vi "USBInterfaceFetch.vi"() -> ()   [LabVIEW 2022 SP3]
uses:
  be0127c4-6358-4ac6-84a7-134a79eb8395.vi
panel:
  in  "Ring":u16(ring) items=["Initialize Pump"=2, "Pump Status"=1, "Interface Only"=0]
  out "read buffer":string
  out "error out":errorcluster
  out "Interface Description":string
  in  "VISA resource name":refnum<visa-resource-name>
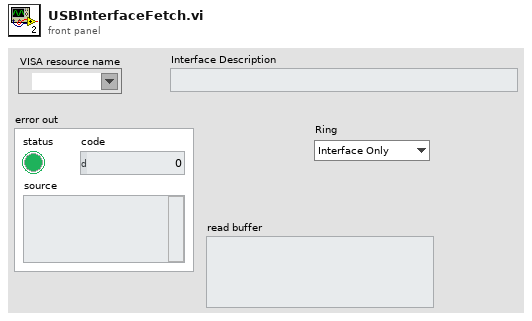
[diagram p1: front panel]
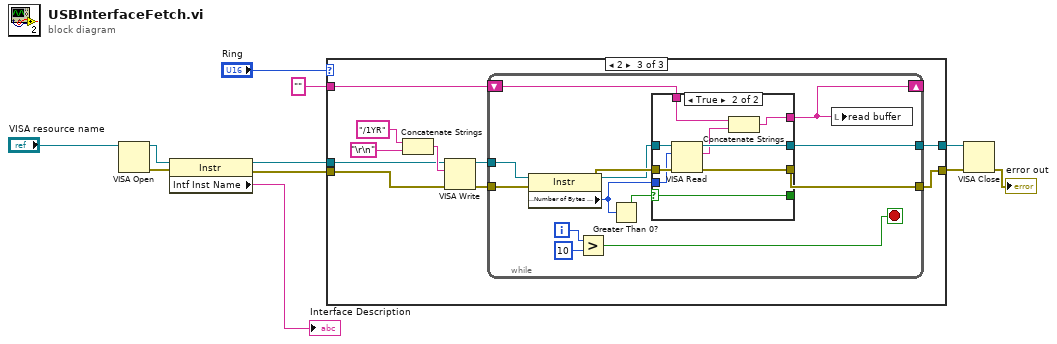
[diagram p0: block diagram]
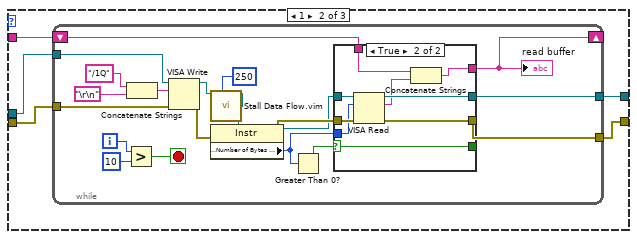
[diagram p3: hidden frame]
diagram:
  n1 = VISA Open(VISA resource name="VISA resource name") -> (VISA resource name=w11:refnum<visa-resource-name>, error out=w9:errorcluster)  [unwired: 4 in]
  n2 = property class="Instr"(reference=w11, error in=w9) -> (reference out=w6:refnum<visa-resource-name>, error out=w8:errorcluster, "Intf Inst Name"=→"Interface Description":string)
  n3 = case shown="2" "Ring" {
    tunnel: w8 -> [w12 w16 w55]
    tunnel: w6 -> [w13 w15 w54]
    tunnel: [w13 w18 w61] -> w4
    tunnel: [w12 w17 w60] -> w3
    tunnel: "" -> [_ w14 w59]
    frame 0, Default {
    }
    frame 1 {
      n4 = while {
        tunnel: [w34] -> w18
        tunnel: [w33] -> w17
        tunnel: w16 -> [w27]
        tunnel: w15 -> [w26]
        shift-right: [w20] -> _
        shift-left: w14 -> [w21]
        i -> [w32]
        stop <- w19 stop-if-true
        n5 = Greater?(x=w32, y=10) -> (0:w19:bool)
        n6 = Concatenate Strings("/1Q" ("write buffer"), "\r\n") -> (w30:string)
        n7 = VISA Write(VISA resource name=w26, write buffer=w30, error in (no error)=w27) -> (VISA resource name out=w23:refnum<visa-resource-name>, error out=w25:errorcluster)  [unwired: 1 out]
        n8 = call "Stall Data Flow.vim"("value in"=w23, "milliseconds to wait"=u32 250) -> ("value out"=w22:refnum<visa-resource-name>)  [unwired: 1 out]
        n9 = property class="Instr"(reference=w22, error in=w25) -> (reference out=w35:refnum<visa-resource-name>, error out=w36:errorcluster, "Serial Settings:Number of Bytes at Serial Port"=w38:u32)
        n10 = Greater Than 0?(x=w38) -> (x > 0?=w37:bool)
        n11 = case shown="True" w37 {
          selector: w37 -> [w40 w46]
          tunnel: w35 -> [w42 w51]
          tunnel: [w42 w50] -> w34
          tunnel: w36 -> [w41 w49]
          tunnel: [w41 w48] -> w33
          tunnel: w38 -> [_ w47]
          tunnel: [w40 w46] -> _
          tunnel: w21 -> [w39 w44]
          tunnel: [w39 w43] -> w20
          frame False {
          }
          frame True {
            n12 = VISA Read(VISA resource name=w51, byte count=w47, error in (no error)=w49) -> (VISA resource name out=w50:refnum<visa-resource-name>, read buffer=w45:string, error out=w48:errorcluster)  [unwired: 1 out]
            n13 = Concatenate Strings(w44, w45) -> (w43:string)
          }
        }
        "read buffer" <- w20
      }
    }
    frame 2 {
      n14 = Concatenate Strings("/1YR" ("write buffer"), "\r\n") -> (w58:string)
      n15 = VISA Write(VISA resource name=w54, write buffer=w58, error in (no error)=w55) -> (VISA resource name out=w52:refnum<visa-resource-name>, error out=w53:errorcluster)  [unwired: 1 out]
      n16 = while {
        tunnel: [w70] -> w61
        tunnel: [w69] -> w60
        shift-right: [w65] -> _
        shift-left: w59 -> [w66]
        tunnel: w53 -> [w64]
        tunnel: w52 -> [w63]
        i -> [w68]
        stop <- w62 stop-if-true
        n17 = property class="Instr"(reference=w63, error in=w64) -> (reference out=w71:refnum<visa-resource-name>, error out=w72:errorcluster, "Serial Settings:Number of Bytes at Serial Port"=w74:u32)
        n18 = Greater?(x=w68, y=10) -> (0:w62:bool)
        n19 = Greater Than 0?(x=w74) -> (x > 0?=w73:bool)
        n20 = case shown="True" w73 {
          selector: w73 -> [w76 w82]
          tunnel: w71 -> [w78 w87]
          tunnel: [w78 w86] -> w70
          tunnel: w72 -> [w77 w85]
          tunnel: [w77 w84] -> w69
          tunnel: w74 -> [_ w83]
          tunnel: [w76 w82] -> _
          tunnel: w66 -> [w75 w80]
          tunnel: [w75 w79] -> w65
          frame False {
          }
          frame True {
            n21 = VISA Read(VISA resource name=w87, byte count=w83, error in (no error)=w85) -> (VISA resource name out=w86:refnum<visa-resource-name>, read buffer=w81:string, error out=w84:errorcluster)  [unwired: 1 out]
            n22 = Concatenate Strings(w80, w81) -> (w79:string)
          }
        }
        n23 = local write "read buffer"(w65) -> ()
      }
    }
  }
  n24 = VISA Close(VISA resource name=w4, error in (no error)=w3) -> (error out=→"error out":errorcluster)
